vi "Ball Intake SS Outputs.vi"(11 "Ball Intake Actuator In":T2) -> (0 "error out":T1)   [LabVIEW 2016]
uses:
  Ball Intake Actuator Out.ctl
  Ball Intake Errors.ctl
  Global Variables/Refnum Names.vi
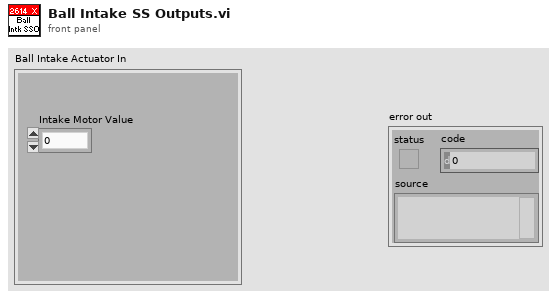
[diagram p1: front panel]
types:
  T1 = typedef "Ball Intake Errors.ctl" = errorcluster
  T2 = typedef "Ball Intake Actuator Out.ctl" = cluster{"Intake Motor Value":dbl}
  T3 = typedef "WPI_MotorControlDeviceRef.ctl" = cluster{"DeviceStatus":errorcluster, "Type":T4, "PWM":cluster{"PWM Channel":T5, "DeadBand":T6}, "CAN":cluster{"Device Number":u8, "SetOutput VI Ref":variant, "GetOutput VI Ref":variant, "Enable VI Ref":variant, "Disable VI Ref":variant, "Data":variant}, "Invert":bool}
  T4 = typedef "WPI_MotorControlType.ctl" = enum16{"PWM", "CAN"}
  T5 = typedef "FPGA_DIOPWMChannel.ctl" = enum8{"PWM 0", "PWM 1", "PWM 2", "PWM 3", "PWM 4", "PWM 5", "PWM 6", "PWM 7", "PWM 8", "PWM 9", "PWM MXP 0", "PWM MXP 1", "PWM MXP 2", "PWM MXP 3", "PWM MXP 4", "PWM MXP 5", "PWM MXP 6", "PWM MXP 7", "PWM MXP 8", "PWM MXP 9", "Invalid"}
  T6 = typedef "WPI_PWMDeadband.ctl" = cluster{"Name":string, "maxPositivePwm":i32, "minPositivePwm":i32, "centerPwm":i32, "maxNegativePwm":i32, "minNegativePwm":i32, "angularRange":u16}
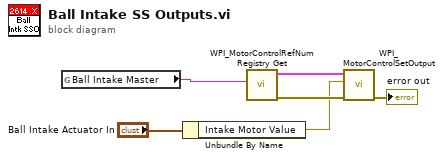
[diagram p0: block diagram]
diagram:
  n1 = global read "Refnum Names.vi" "Ball Intake Master"() -> (w5:string)
  n2 = Unbundle By Name("Ball Intake Actuator In") -> ("Intake Motor Value"=w1:dbl)
  n3 = call <vilib>:"WPI_MotorControlRefNum Registry Get.vi"("refnum name"=w5) -> ("error out"=w4:errorcluster, "MotorControlDevRef"=w2:T3)  [unwired: 9 in]
  n4 = call <vilib>:"WPI_MotorControlSetOutput.vi"("error in (no error)"=w4, "Output"=w1, "MotorControlDevRef"=w2) -> ("error out"=→"error out":errorcluster)  [unwired: 6 in, 2 out]
